vi "PathPlanner_RotationTarget_Flip.vi"(11 "RotationTarget":T1={"position"=0.0, "rotation"={"VALUE"=0.0, "COS"=1.0, "SIN"=0.0}, "Exists"=FALSE} {"rotation"."SIN" format="%13.4f"; "rotation"."COS" format="%13.4f"; "rotation"."VALUE" format="%13.4f"}) -> (3 "FlippedRotationTarget":T1={"position"=0.0, "rotation"={"VALUE"=0.0, "COS"=1.0, "SIN"=0.0}, "Exists"=FALSE} {"rotation"."SIN" format="%13.4f"; "rotation"."COS" format="%13.4f"; "rotation"."VALUE" format="%13.4f"})   [LabVIEW 2019, in "PathPlanner24.lvlib"]
doc: "Flip a rotation target for the other side of the field, maintaining a blue alliance origin\n\nInputs: \n - RotationTarget - cluster - defined rotation target data structure\n \nOutputs:\n - FlippedRotationTarget - cluster - The flipped rotation target"
uses:
  PathPlanner24.lvlib
  TypeDef/PathPlannerRotationTarget.ctl
  <vilib>/Rock Robotics/WPI/ThirdParty/JAS_Junk/TrajLib/TypeDef/ROTATION2D.ctl
  PathPlanner_FieldUtil_SymmetryType.vi
  <vilib>/Rock Robotics/WPI/ThirdParty/JAS_Junk/TrajLib/Rotation2d_CreateAngle.vi
  <vilib>/Rock Robotics/WPI/ThirdParty/JAS_Junk/TrajLib/Rotation2d_Minus.vi
  <vilib>/Rock Robotics/WPI/ThirdParty/JAS_Junk/TrajLib/Rotation2d_UnaryMinus.vi
  <vilib>/Rock Robotics/WPI/ThirdParty/JAS_Junk/TrajLib/Rotation2d_RotateBy.vi
  <vilib>/Rock Robotics/WPI/ThirdParty/JAS_Junk/TrajLib/Rotation2d_CreateXY.vi
  <vilib>/Rock Robotics/WPI/ThirdParty/JAS_Junk/TrajLib/Util_CalcDist.vi
  <vilib>/Rock Robotics/WPI/ThirdParty/JAS_Junk/TrajLib/Trajectory_Library.lvlib
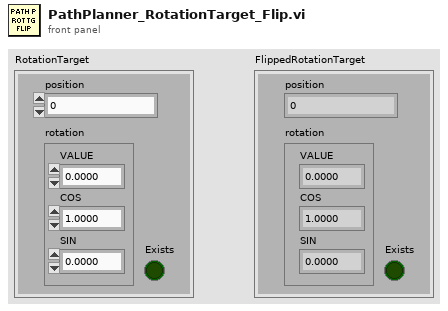
[diagram p1: front panel]
types:
  T1 = typedef "PathPlanner24.lvlib/PathPlannerRotationTarget.ctl" = cluster{"position":dbl, "rotation":T2, "Exists":bool}
  T2 = typedef "Trajectory_Library.lvlib/ROTATION2D.ctl" = cluster{"VALUE":dbl, "COS":dbl, "SIN":dbl}
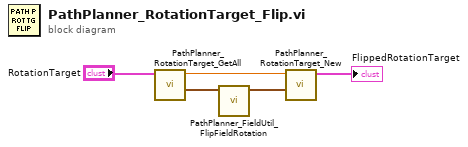
[diagram p0: block diagram]
diagram:
  n1 = call "PathPlanner_RotationTarget_GetAll.vi"("RotationTarget"="RotationTarget") -> ("rotation"=w3:T2, "position"=w4:dbl)  [unwired: 8 in, 1 out]
  n2 = call "PathPlanner_FieldUtil_FlipFieldRotation.vi"("rotation"=w3) -> ("flippedRotation"=w2:T2)  [unwired: 10 in]
  n3 = call "PathPlanner_RotationTarget_New.vi"("rotation"=w2, "position"=w4) -> ("RotationTarget"=→"FlippedRotationTarget":T1)  [unwired: 9 in]
